vi "题目1.vi"() -> ()   [LabVIEW 2017]
uses:
  <vilib>/measure/NI_MABase.lvlib
panel:
  in  "开关":bool
  out "方波":waveform(dbl)(graph)
  out "正弦波":waveform(dbl)(graph)
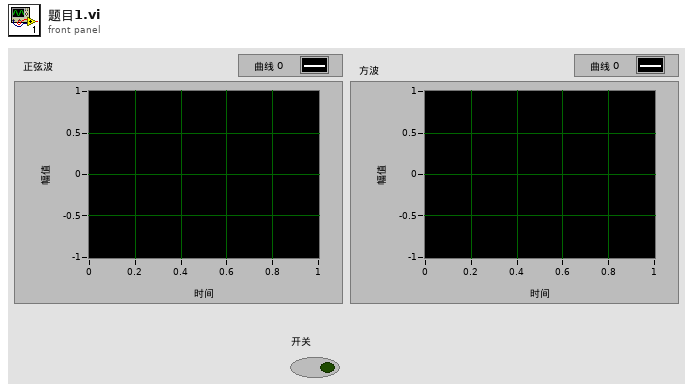
[diagram p1: front panel]
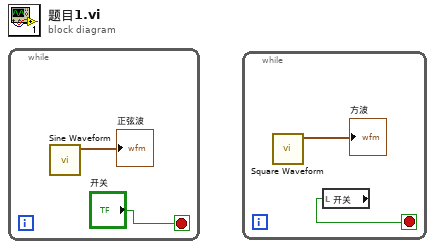
[diagram p0: block diagram]
diagram:
  n1 = while {
    stop <- "开关" stop-if-true
    n2 = call <vilib>:"Sine Waveform.vi"() -> ("signal out"=→"正弦波":waveform(dbl))  [unwired: 10 in, 1 out]
  }
  n3 = while {
    stop <- w3 stop-if-true
    n4 = call <vilib>:"Square Waveform.vi"() -> ("signal out"=→"方波":waveform(dbl))  [unwired: 10 in, 1 out]
    n5 = local read "开关"() -> (w3:bool)
  }
